vi "Vi 3.vi"() -> ()   [LabVIEW 2010]
panel:
  in  "Slide":dbl(slide) scale=0.0..10.0
  in  "stop":bool
  out "Area del cìrculo":dbl
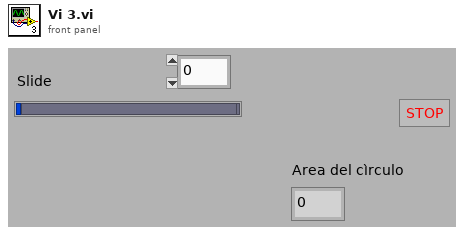
[diagram p1: front panel]
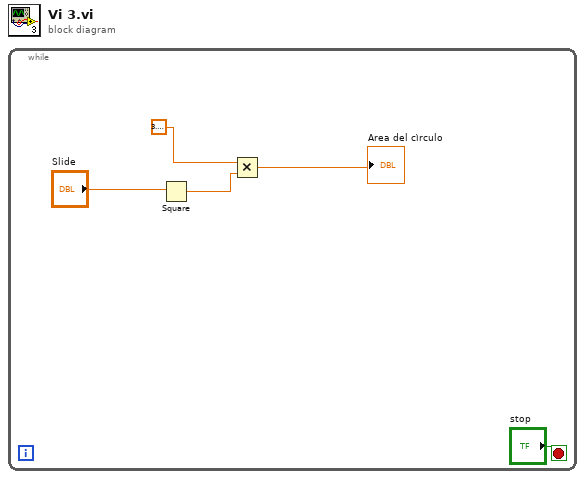
[diagram p0: block diagram]
diagram:
  n1 = while {
    stop <- "stop" stop-if-true
    n2 = Square(x="Slide") -> (x^2=w3:dbl)
    n3 = Multiply(x=3.141592653589793, y=w3) -> (x*y=→"Area del cìrculo":dbl)
  }
